vi "Get PING))) Sensor.vi"(8 "error in (no error)":errorcluster, 11 "NI_Robotics_Starter Kit Host in":refnum<class "NI_Robotics_Starter Kit Host.lvclass">) -> (0 "error out":errorcluster, 2 "PING)))":refnum<class "Parallax PING))).lvclass">, 3 "NI_Robotics_Starter Kit Host out":refnum<class "NI_Robotics_Starter Kit Host.lvclass">)   [LabVIEW 2017, in "NI_Robotics_Starter Kit Host.lvclass"]
uses:
  <vilib>/robotics/Starter Kit/Host Interface/NI_Robotics_Starter Kit Host.lvclass
  <instrlib>/Parallax PING)))/HAIOL/Parallax PING))).lvclass
  <vilib>/robotics/Starter Kit/Host Interface/NI_Robotics_Starter Kit Host.lvclass/NI_Robotics_Starter Kit Host.ctl
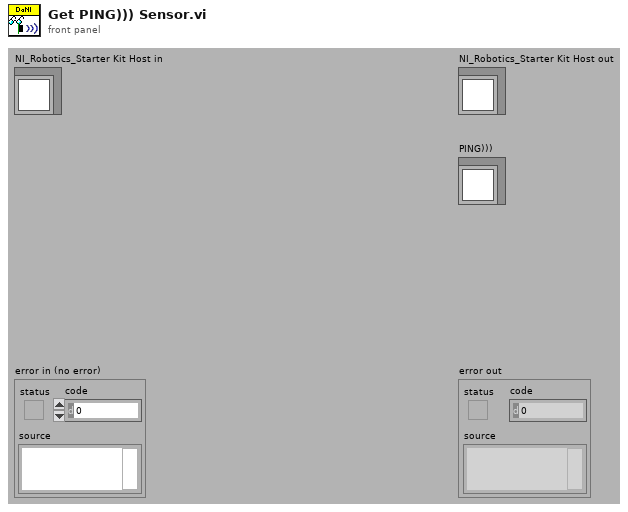
[diagram p1: front panel]
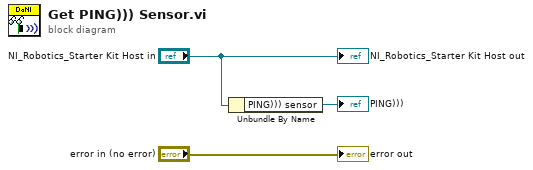
[diagram p0: block diagram]
diagram:
  n1 = Unbundle By Name("NI_Robotics_Starter Kit Host in") -> ("PING))) sensor"=→"PING)))":refnum<class "Parallax PING))).lvclass">)
  "error out" <- "error in (no error)"
  "NI_Robotics_Starter Kit Host out" <- "NI_Robotics_Starter Kit Host in"
